vi "RST.vi"(8 "error in (no error)":errorcluster, 11 "Reference in":T1={"Device"="", "Function"="", "delay"=20}) -> (0 "error out":errorcluster, 3 "Reference out":T1={"Device"="", "Function"="", "delay"=20})   [LabVIEW 2021, in "Rigol DM3052.lvlib"]
uses:
  Rigol DM3052.lvlib
  Reference.ctl
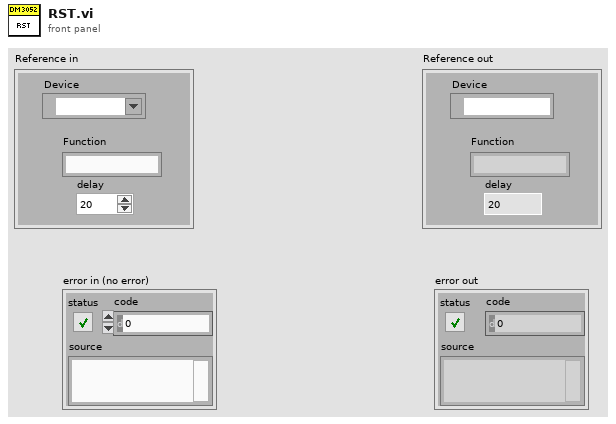
[diagram p1: front panel]
types:
  T1 = typedef "Rigol DM3052.lvlib/Reference.ctl" = cluster{"Device":refnum<visa-resource-name>, "Function":string, "delay":u32}
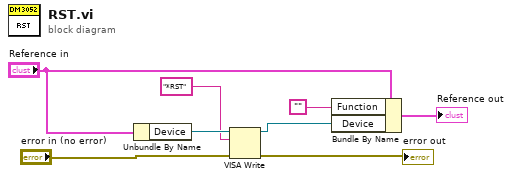
[diagram p0: block diagram]
diagram:
  n1 = Unbundle By Name("Reference in") -> ("Device"=w4:refnum<visa-resource-name>)
  n2 = VISA Write(VISA resource name=w4, write buffer="*RST", error in (no error)="error in (no error)") -> (VISA resource name out=w5:refnum<visa-resource-name>, error out=→"error out":errorcluster)  [unwired: 1 out]
  n3 = Bundle By Name(cluster="Reference in", "Function"="", "Device"=w5) -> (→"Reference out":T1)
